vi "basic-delay.vi"(0 "Cluster in":refnum<vi>, 1 "reference in":refnum<vi>, 2 "Numeric":dbl, 3 "Current Number Delay Licks":i32, 5 "Lickometer":refnum<vi>, 7 "Cluster 3":T1, 9 "Period":i64, 12 "relative seconds":dbl, 13 "Min Licks":i32, 14 "Cluster 2":T2) -> (4 "Cluster 4":T1, 6 "Cluster":T2)   [LabVIEW 2015]
uses:
  <vilib>/Platform/TimedLoop/XDataNode/wakeup.ctl
  <vilib>/Platform/TimedLoop/XDataNode/XDNodeRunTimeDep.lvlib
  <vilib>/Platform/TimedLoop/XDataNode/nitl_modes.ctl
  <vilib>/Platform/TimedLoop/XDataNode/timing_clust.ctl
  <vilib>/platform/TimedLoop/XDataNode/XDataNode.xnode
  Device/Methods/Lickometer-Read.vi
  Rack/Methods/Rack-Refresh.vi
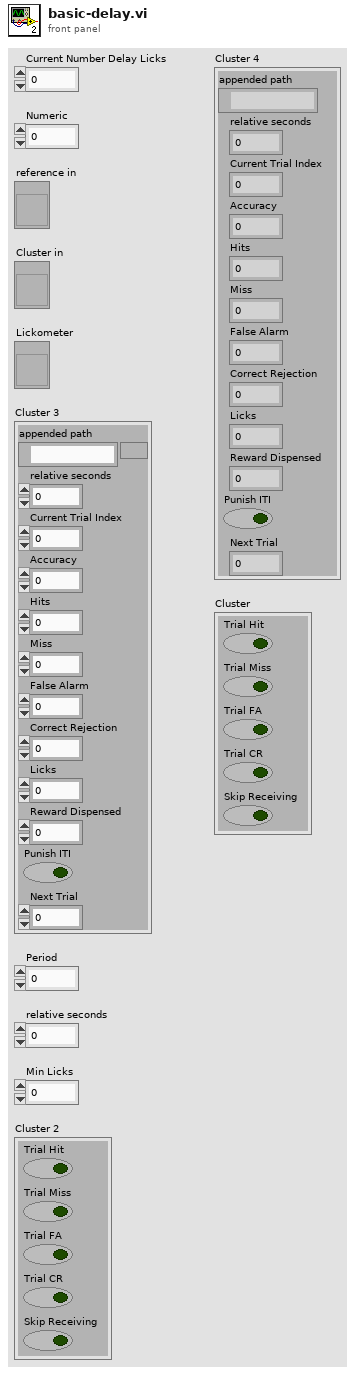
[diagram p1: front panel]
types:
  T1 = cluster{"appended path":path, "relative seconds":dbl, "Current Trial Index":i32, "Accuracy":dbl, "Hits":i32, "Miss":i32, "False Alarm":i32, "Correct Rejection":i32, "Licks":i32, "Reward Dispensed":dbl, "Punish ITI":bool, "Next Trial":i32}
  T2 = cluster{"Trial Hit":bool, "Trial Miss":bool, "Trial FA":bool, "Trial CR":bool, "Skip Receiving":bool}
  T3 = typedef "XDNodeRunTimeDep.lvlib/timing_clust.ctl" = cluster{"Expected End [f-1]":u64, "Actual End [f-1]":u64, "Finished Late? [f-1]":bool, "Expected End [i-1]":u64, "Actual End [i-1]":u64, "Finished Late? [i-1]":bool, "Expected Start [i]":u64, "Actual Start [i]":u64, "Expected Start [f]":u64, "Actual Start [f]":u64, "Source Name":string, "Structure Name":string, "Period":i64, "Deadline":i64, "Offset":i64, "Start":i64, "Priority":i32, "Timeout":i32, "Mode":T4, "Wakeup Reason":T5, "Error":errorcluster, "Source Type":string, "Secondary Source Type":string, "Global End Time":u64, "Global Start Time":u64, "Frame Duration":u64, "Iteration Duration":u64, "Assigned CPU":i32, "I/O Scan Engine Mode":u32}
  T4 = typedef "XDNodeRunTimeDep.lvlib/nitl_modes.ctl" = enum32{"No Change", "Process missed periods, maintain original phase", "Discard missed periods, maintain original phase", "Process missed periods, ignore original phase", "Discard missed periods, ignore original phase"}
  T5 = typedef "XDNodeRunTimeDep.lvlib/wakeup.ctl" = enum32{"Normal", "Aborted", "Asynchronous wakeup", "Timing source error", "Timed loop error", "Timeout"}
  T6 = typedef "InputData cluster.ctl" = cluster{"DigitalInput":T7}
  T7 = typedef "DigitalInput-DataCluster.ctl" = cluster{"Falling":bool[], "Rising":bool[], "State":bool[]}
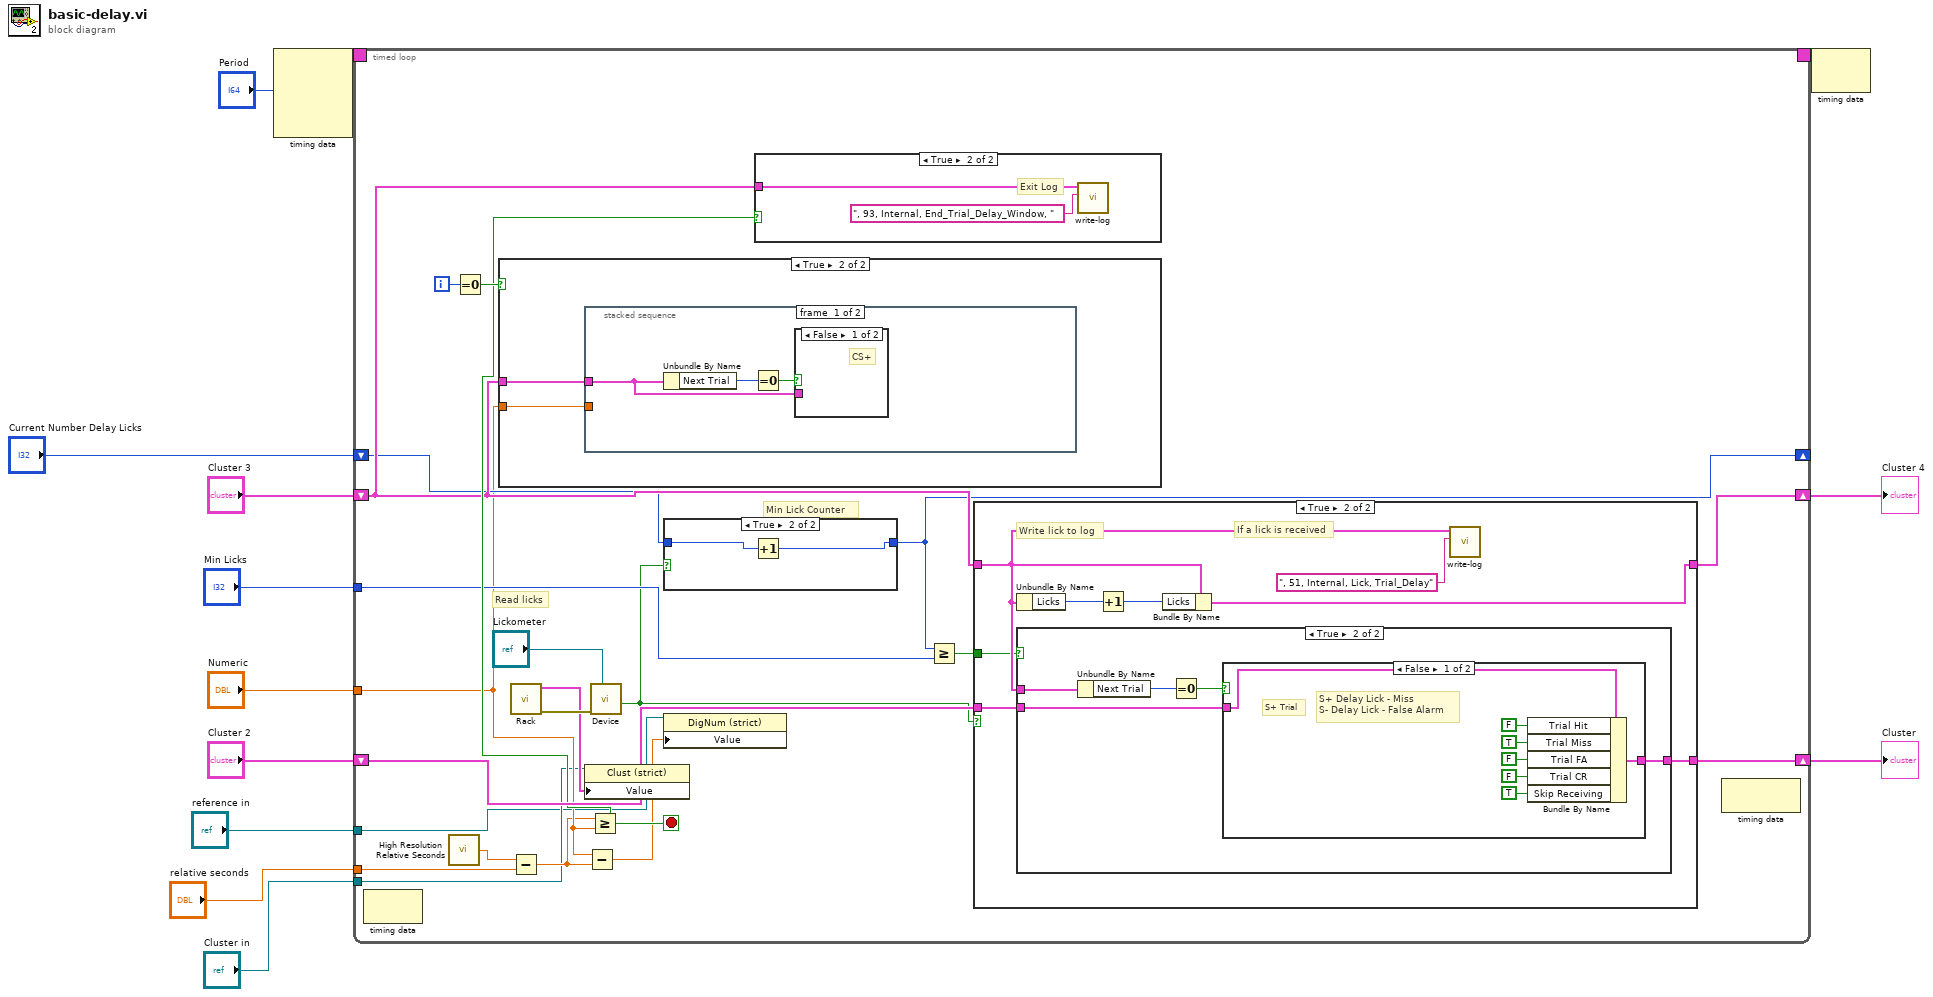
[diagram p0: block diagram]
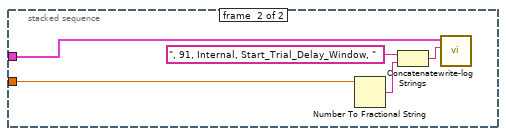
[diagram p6: hidden frame]
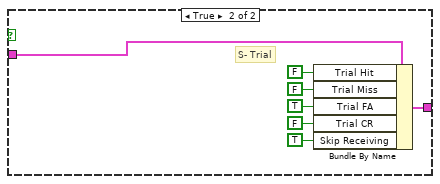
[diagram p9: hidden frame]
diagram:
  n1 = node-c288("Period") -> (w13:T3)  [unwired: 3 in]
  n2 = timed-loop {
    tunnel: "Numeric" -> [w18]
    tunnel: "relative seconds" -> [w33]
    shift-right: [w34] -> w4
    shift-left: "Cluster 3" -> [w27]
    shift-right: [w31] -> w7
    shift-left: "Cluster 2" -> [w32]
    tunnel: "Min Licks" -> [w23]
    shift-right: [w25] -> _
    shift-left: "Current Number Delay Licks" -> [w26]
    timing: w13 -> [_]
    timing-out: [_] -> w12
    tunnel: "Cluster in" -> [w15]
    tunnel: "reference in" -> [w14]
    i -> [w30]
    stop <- w28 stop-if-true
    # "Min Lick Counter"
    # "Read licks"
    n3 = node-c288() -> ()  [unwired: 1 in, 1 out]
    n4 = call <vilib>:"High Resolution Relative Seconds.vi"() -> ("relative seconds"=w35:dbl)
    n5 = Equal To 0?(x=w30) -> (x = 0?=w29:bool)
    n6 = case shown="True" w29 {
      tunnel: w27 -> [_ w43]
      tunnel: w18 -> [_ w44]
      frame False {
      }
      frame True {
        n7 = stacked-sequence {
          tunnel: w44 -> [_ w48]
          tunnel: w43 -> [w46 w49]
          frame #0 {
            n8 = Unbundle By Name(w46) -> ("Next Trial"=w47:i32)
            n9 = Equal To 0?(x=w47) -> (x = 0?=w45:bool)
            n10 = case shown="False" w45 {
              tunnel: w46 -> [_ _]
              frame False {
                # "CS+"
              }
              frame True {
                # "CS-"
              }
            }
          }
          frame #1 {
            n11 = Number To Fractional String(number=w48) -> (F-format string=w50:string)  [unwired: 3 in]
            n12 = Concatenate Strings(", 91, Internal, Start_Trial_Delay_Window, " ("text"), w50) -> (w51:string)
            n13 = call "write-log.vi"("Write Text"=w51, "Internal Cluster"=w49) -> ()  [unwired: 10 in]
          }
        }
      }
    }
    n14 = call-poly "Rack.vi"() -> ("error out"=w21:errorcluster, "Data Cluster"=w19:T6)  [unwired: 10 in]
    n15 = Subtract(x=w35, y=w33) -> (x-y=w17:dbl)
    n16 = property class="Clust (strict)"(reference=w15, "Value"=w19) -> ()  [unwired: 1 in, 2 out]
    n17 = Subtract(x=w18, y=w17) -> (x-y=w16:dbl)
    n18 = Greater Or Equal?(x=w17, y=w18) -> (x >= y?=w28:bool)
    n19 = call-poly "Device.vi"("Device reference"="Lickometer", "error in (no error)"=w21) -> ("Lick start?"=w22:bool)  [unwired: 7 in, 2 out]
    n20 = case shown="True" w22 {
      tunnel: w26 -> [w38 w40]
      tunnel: [w38 w39] -> w25
      frame False {
      }
      frame True {
        n21 = Increment(x=w40) -> (x+1=w39:i32)
      }
    }
    n22 = property class="DigNum (strict)"(reference=w14, "Value"=w16) -> ()  [unwired: 1 in, 2 out]
    n23 = case shown="True" w28 {
      tunnel: w27 -> [_ w42]
      frame False {
      }
      frame True {
        # "Exit Log"
        n24 = call "write-log.vi"("Write Text"=", 93, Internal, End_Trial_Delay_Window, " ("text"), "Internal Cluster"=w42) -> ()  [unwired: 10 in]
      }
    }
    n25 = Greater Or Equal?(x=w25, y=w23) -> (x >= y?=w24:bool)
    n26 = case shown="True" w22 {
      tunnel: w27 -> [w54 w58]
      tunnel: [w54 w59] -> w34
      tunnel: w32 -> [w53 w57]
      tunnel: [w53 w56] -> w31
      tunnel: w24 -> [_ w55]
      frame False {
      }
      frame True {
        # "If a lick is received"
        # "Write lick to log"
        n27 = Unbundle By Name(w58) -> ("Licks"=w61:i32)
        n28 = case shown="True" w55 {
          tunnel: w58 -> [_ w68]
          tunnel: w57 -> [w63 w65]
          tunnel: [w63 w64] -> w56
          frame False {
          }
          frame True {
            n29 = Unbundle By Name(w68) -> ("Next Trial"=w67:i32)
            n30 = Equal To 0?(x=w67) -> (x = 0?=w66:bool)
            n31 = case shown="False" w66 {
              tunnel: w65 -> [w71 w82]
              tunnel: [w69 w79] -> w64
              frame False {
                # "S+ Delay Lick - Miss\nS- Delay Lick - False Alarm"
                # "S+ Trial"
                n32 = Bundle By Name(cluster=w71, "Trial Hit"=FALSE ("Trial FA"), "Trial Miss"=TRUE ("Trial CR"), "Trial FA"=FALSE ("Trial CR"), "Trial CR"=FALSE, "Skip Receiving"=TRUE) -> (w69:T2)
              }
              frame True {
                # "S- Trial"
                n33 = Bundle By Name(cluster=w82, "Trial Hit"=FALSE ("Trial FA"), "Trial Miss"=FALSE ("Trial CR"), "Trial FA"=TRUE ("Trial CR"), "Trial CR"=FALSE, "Skip Receiving"=TRUE) -> (w79:T2)
              }
            }
          }
        }
        n34 = Increment(x=w61) -> (x+1=w60:i32)
        n35 = Bundle By Name(cluster=w58, "Licks"=w60) -> (w59:T1)
        n36 = call "write-log.vi"("Write Text"=", 51, Internal, Lick, Trial_Delay" ("text"), "Internal Cluster"=w58) -> ()  [unwired: 10 in]
      }
    }
    n37 = node-c288() -> ()  [unwired: 1 in, 1 out]
  }
  "Cluster" <- w7
  "Cluster 4" <- w4
  n38 = node-c288(w12) -> ()  [unwired: 1 out]
